vi "find data server.vi"(11 "Data Servers":string[](array[string])=["enviro.cee.cornell.edu", "calcium.cee.cornell.edu"]) -> (0 "Restart":bool, 2 "Data Servers out":string[](array[string])=["calcium", "Dataserver"], 3 "data server address out":string="128.84.245.227")   [LabVIEW 2012]
panel:
  in  "Okay":bool
  in  "Restart":bool
  # "Choose the data server by changing the array index or by typing an IP address into one of the array elements.\n\n\nIf you have trouble connecting:\nVerify that the data server is running and then RESTART this program\nsoftware."
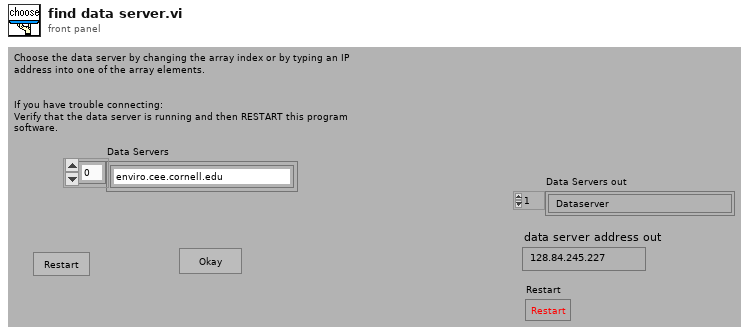
[diagram p1: front panel]
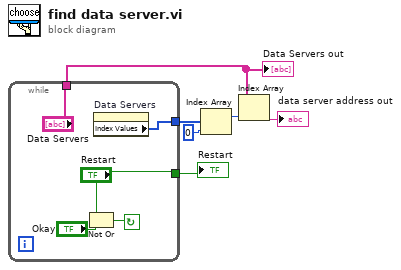
[diagram p0: block diagram]
diagram:
  n1 = while {
    tunnel: [w7] -> w4
    tunnel: ["Data Servers"] -> w1
    tunnel: ["Restart"] -> w6
    stop <- w10 continue-if-true
    n2 = Not Or(1:"Okay", 2:"Restart") -> (0:w10:bool)
    n3 = property on="Data Servers" class="Arr (strict)"() -> ("Index Values"=w7:u32[])  [unwired: 2 in, 2 out]
  }
  "Restart" <- w6
  "Data Servers out" <- w1
  n4 = Index Array(array=w4, index=0 ("Index")) -> (element=w2:u32)
  n5 = Index Array(array=w1, index=w2) -> (element=→"data server address out":string)
